vi "rs3 get video stream resolution.vi"(8 "error in (no error)":errorcluster, 11 "Profile":u64) -> (0 "error out":errorcluster, 1 "height":u32, 2 "width":u32, 3 "Profile out":u64, 5 "error":u64)   [LabVIEW 2019, in "libRealSense3.lvlib"]
doc: "Returns the (X,Y) resolution of a specific PROFILE."
uses:
  libRealSense3.lvlib
  realsense2.dll
panel:
  # "RS3 Get Stream Resolution"
  # "(C) Intel Corp.,  AGJ 2017"
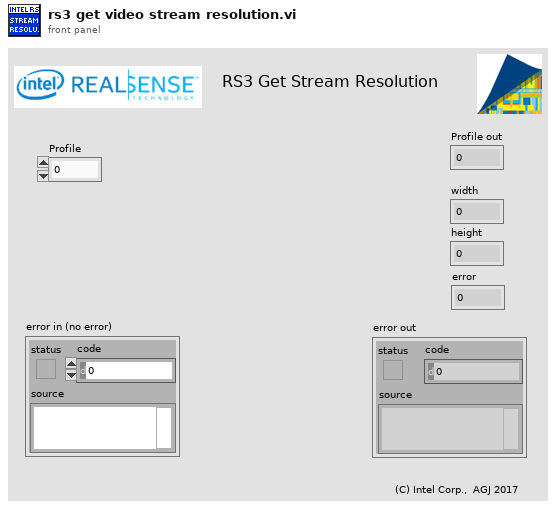
[diagram p1: front panel]
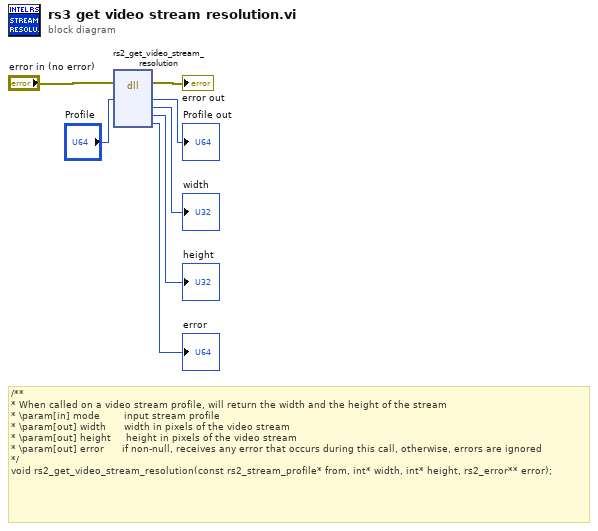
[diagram p0: block diagram]
diagram:
  # "/**\n* When called on a video stream profile, will return the width and the height of the stream\n* \\param[in] mode        input stream profile\n* \\param[out] width      width in pixels of the video stream\n* \\param[out] height     height in pixels of the video stream\n* \\param[out] error      if non-null, receives any error that occurs during this call, otherwise, errors are ignored\n*/\nvoid rs2_get_video_stream_resolution(const rs2_stream_profile* from, int* width, int* height, rs2_error** error);"
  n1 = dll-call lib="C:/Users/morte/Documents/gitmoro/treadmill/RealSense for Labview ver. 2.33/realsense2.dll" fn="rs2_get_video_stream_resolution"(error in="error in (no error)", "Profile"="Profile") -> (error out=→"error out":errorcluster, "Profile"=→"Profile out":u64, "width"=→"width":u32, "height"=→"height":u32, "error"=→"error":u64)  [unwired: 6 in, 1 out]
